vi "Capacitive Message Loop.vi"(8 "error in (no error)":errorcluster, 10 "Data Notifiers":T1, 11 "Message Queues":T2) -> (0 "error out":errorcluster)   [LabVIEW 2013, in "Capacitive.lvlib"]
uses:
  Capacitive.lvlib
  support/Message Queue/All Message Queues.ctl
  support/Message Queue/Message Cluster.ctl
  support/Data Notifiers/All Data Notifiers.ctl
  Acquisition/APD Notifier Cluster.ctl
  Piezo/Piezo display.ctl
  XY/XY Display.ctl
  Capacitive Signal Cluster.ctl
  Hardware Configuration.ctl
  Acquisition/Acquisition State.ctl
  support/Message Queue/Enqueue Message (Single).vi
  <vilib>/Utility/error.llb/Error Cluster From Error Code.vi
  <vilib>/ErrorRing/Error Ring.xnode
  Acquisition/Acquisition.lvlib
  support/Message Queue/Message Queue.lvlib
  Piezo/Piezo.lvlib
  XY/XY.lvlib
  support/Data Notifiers/Data Notifiers.lvlib
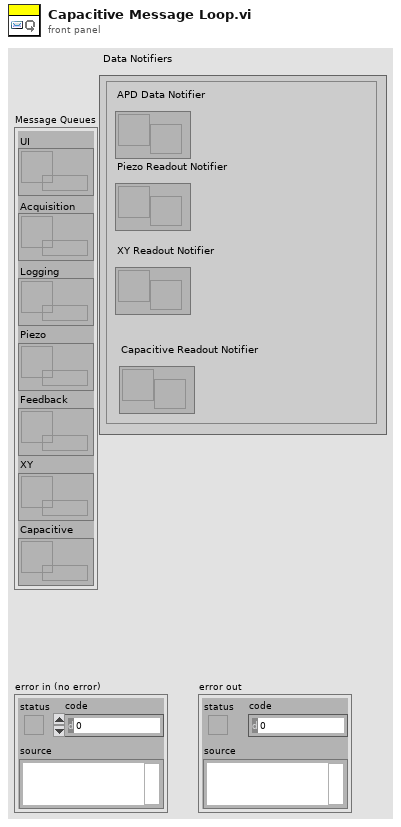
[diagram p1: front panel]
types:
  T1 = typedef "Data Notifiers.lvlib/All Data Notifiers.ctl" = cluster{"APD Data Notifier":refnum<notifier>, "Piezo Readout Notifier":refnum<notifier>, "XY Readout Notifier":refnum<notifier>, "Capacitive Readout Notifier":refnum<notifier>}
  T2 = typedef "Message Queue.lvlib/All Message Queues.ctl" = cluster{"UI":refnum<queue>, "Acquisition":refnum<queue>, "Logging":refnum<queue>, "Piezo":refnum<queue>, "Feedback":refnum<queue>, "XY":refnum<queue>, "Capacitive":refnum<queue>}
  T3 = typedef "Capacitive.lvlib/Hardware Configuration.ctl" = cluster{"IP Address":string, "Handle":u32, "Refresh Time (ms)":dbl}
  T4 = typedef "Acquisition.lvlib/Acquisition State.ctl" = enum16{"Idle", "Acquiring"}
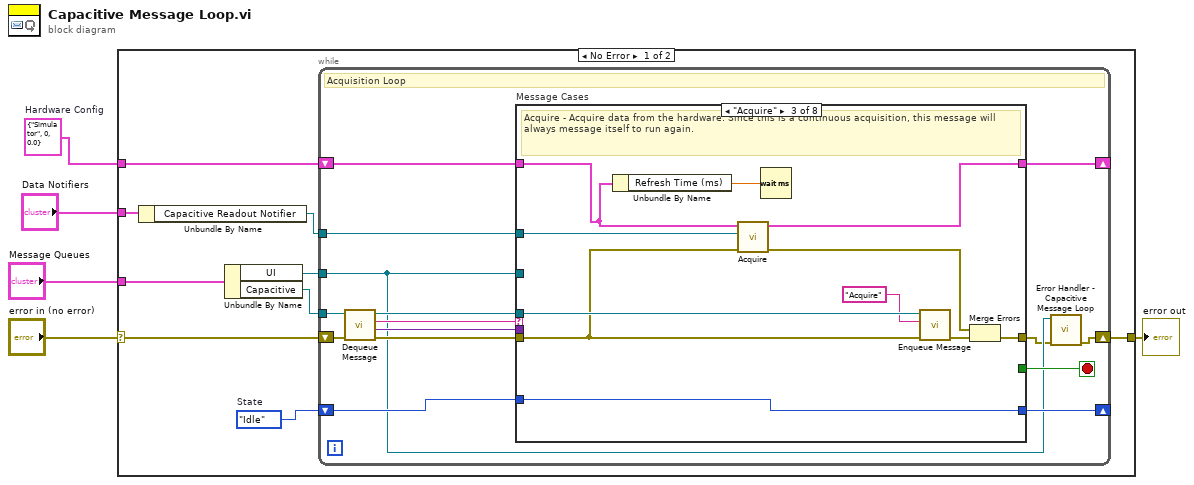
[diagram p0: block diagram]
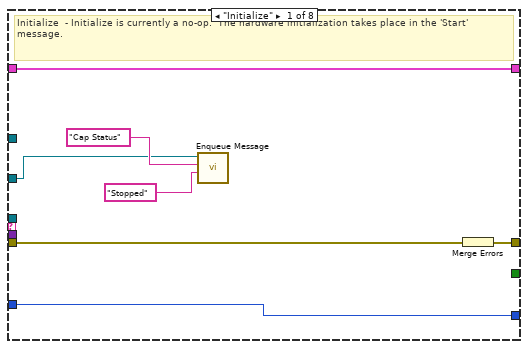
[diagram p2: hidden frame]
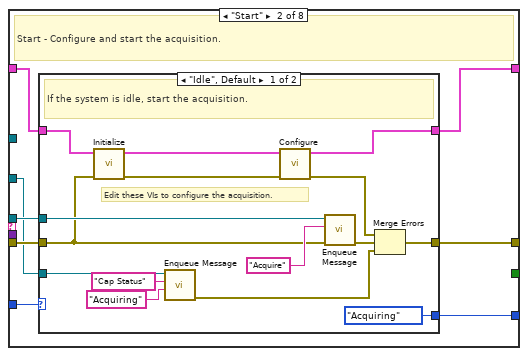
[diagram p3: hidden frame]
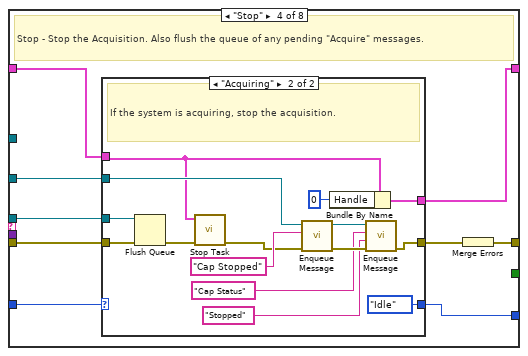
[diagram p5: hidden frame]
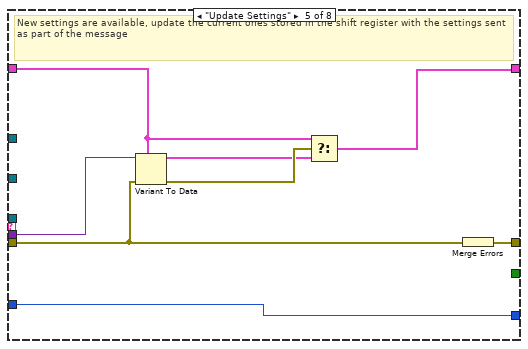
[diagram p7: hidden frame]
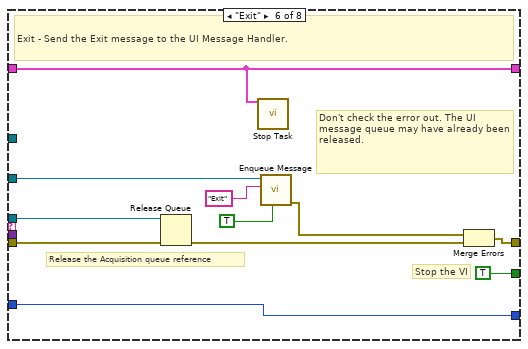
[diagram p8: hidden frame]
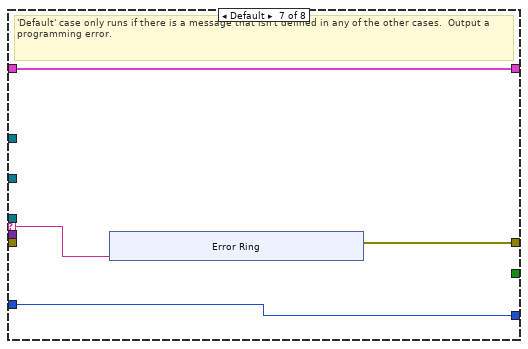
[diagram p9: hidden frame]
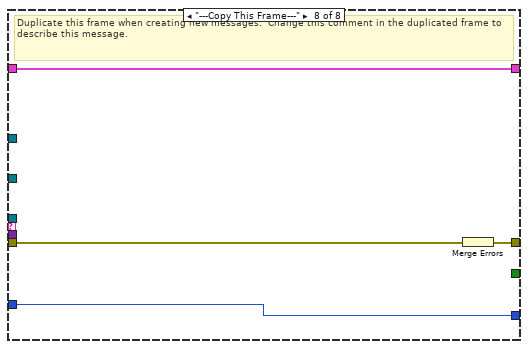
[diagram p10: hidden frame]
diagram:
  w2 = T3 {"IP Address"="Simulator", "Handle"=0, "Refresh Time (ms)"=0.0}  # Hardware Config
  n1 = case shown="No Error" "error in (no error)" {
    selector: "error in (no error)" -> [w11 w135]
    tunnel: "Message Queues" -> [w14 _]
    tunnel: [w12 w135] -> w4
    tunnel: w2 -> [w8 _]
    tunnel: "Data Notifiers" -> [w7 _]
    frame No Error {
      w9 = Acquisition_State."Idle"  # State
      n2 = Unbundle By Name(w7) -> ("Capacitive Readout Notifier"=w6:refnum<notifier>)
      n3 = Unbundle By Name(w14) -> ("UI"=w10:refnum<queue>, "Capacitive"=w13:refnum<queue>)
      n4 = while {
        tunnel: w13 -> [w21]
        shift-right: [w28] -> _
        shift-left: w8 -> [w29]
        shift-right: [w15] -> w12
        shift-left: w11 -> [w26]
        tunnel: w10 -> [w17]
        shift-right: [w19] -> _
        shift-left: w9 -> [w20]
        tunnel: w6 -> [w18]
        stop <- w27 stop-if-true
        # "Acquisition Loop"
        n5 = call "Dequeue Message.vi"("error in (no error)"=w26, "Message Queue"=w21) -> ("error out"=w25:errorcluster, "Message Data"=w23:variant, "Message"=w24:string, "dup Message Queue"=w22:refnum<queue>)  [unwired: 6 in]
        n6 = case "Message Cases" shown="\"Acquire\"" w24 {
          selector: w24 -> [_ _ _ _ _ _ w122 _]
          tunnel: w22 -> [_ w41 w71 w79 _ w112 _ _]
          tunnel: w25 -> [w35 w42 w67 w81 w102 w116 _ w134]
          tunnel: [w36 w44 w73 w82 w108 w118 w121 w132] -> w16
          tunnel: w29 -> [w34 w43 w64 w80 w104 w110 w123 w133]
          tunnel: [w34 w40 w68 w74 w103 w110 w123 w133] -> w28
          tunnel: [_ _ _ _ _ TRUE _ _] -> w27
          tunnel: w23 -> [_ _ _ _ w107 _ _ _]
          tunnel: w17 -> [w30 w37 _ w78 _ w117 _ _]
          tunnel: w20 -> [w33 w39 w69 w77 w101 w111 w120 w131]
          tunnel: [w33 w38 w69 w76 w101 w111 w120 w131] -> w19
          tunnel: w18 -> [_ _ w65 _ _ _ _ _]
          frame "Initialize" {
            # "Initialize  - Initialize is currently a no-op.  The hardware initialization takes place in the 'Start' message."
            n7 = call-poly "Enqueue Message.vi"("Message Data"="Stopped" ("Message"), "Message"="Cap Status", "Message Queue"=w30) -> ()  [unwired: 7 in, 2 out]
            n8 = Merge Errors(w35) -> (w36:errorcluster)
          }
          frame "Start" {
            # "Start - Configure and start the acquisition."
            n9 = case shown="\"Idle\", Default" w39 {
              selector: w39 -> [_ w60]
              tunnel: [w59 w62] -> w44
              tunnel: w43 -> [w53 w61]
              tunnel: w42 -> [w54 w62]
              tunnel: w41 -> [w57 _]
              tunnel: [w51 w61] -> w40
              tunnel: [Acquisition_State."Acquiring" ("State") w60] -> w38
              tunnel: w37 -> [w47 _]
              frame "Idle", Default {
                # "Edit these VIs to configure the acquisition."
                # "If the system is idle, start the acquisition."
                n10 = call "Initialize.vi"("error in (no error)"=w54, "Hardware Refs In"=w53) -> ("error out"=w50:errorcluster, "Hardware Refs Out"=w52:T3)  [unwired: 8 in]
                n11 = call-poly "Enqueue Message.vi"("Message Data"="Acquiring" ("Message"), "Message"="Cap Status", "Message Queue"=w47) -> ("error out"=w48:errorcluster)  [unwired: 7 in, 1 out]
                n12 = call "Configure.vi"("error in (no error)"=w50, "Hardware Refs In"=w52) -> ("error out"=w49:errorcluster, "Hardware Refs Out"=w51:T3)  [unwired: 8 in]
                n13 = call-poly "Enqueue Message.vi"("error in (no error)"=w54, "Message"="Acquire", "Message Queue"=w57) -> ("error out"=w58:errorcluster)  [unwired: 7 in, 1 out]
                n14 = Merge Errors(w49, w58, w48) -> (w59:errorcluster)
              }
              frame "Acquiring" {
                # "The system is already acquiring. Ignore the \"Start\" message."
              }
            }
          }
          frame "Acquire" {
            # "Acquire - Acquire data from the hardware. Since this is a continuous acquisition, this message will always message itself to run again."
            n15 = Unbundle By Name(w64) -> ("Refresh Time (ms)"=w63:dbl)
            n16 = call "Acquire.vi"("error in (no error)"=w67, "Capacitive Readout Notifier"=w65, "Hardware Refs In"=w64) -> ("error out"=w66:errorcluster, "Hardware Refs Out"=w68:T3)  [unwired: 7 in]
            n17 = Wait (ms)(milliseconds to wait=w63) -> ()  [unwired: 1 out]
            n18 = call-poly "Enqueue Message.vi"("error in (no error)"=w67, "Message"="Acquire", "Message Queue"=w71) -> ("error out"=w72:errorcluster)  [unwired: 7 in, 1 out]
            n19 = Merge Errors(w66, w72) -> (w73:errorcluster)
          }
          frame "Stop" {
            # "Stop - Stop the Acquisition. Also flush the queue of any pending \"Acquire\" messages."
            n20 = case shown="\"Acquiring\"" w77 {
              selector: w77 -> [w85 _]
              tunnel: w81 -> [w84 w100]
              tunnel: w80 -> [w83 w93]
              tunnel: w79 -> [_ w99]
              tunnel: w78 -> [_ w98]
              tunnel: [w85 Acquisition_State."Idle" ("State")] -> w76
              tunnel: [w84 w89] -> w75
              tunnel: [w83 w91] -> w74
              frame "Idle", Default {
                # "The system is already idle. Ignore the \"Stop\" message."
              }
              frame "Acquiring" {
                # "If the system is acquiring, stop the acquisition."
                n21 = Flush Queue(queue=w99, error in (no error)=w100) -> (error out=w95:errorcluster)  [unwired: 2 out]
                n22 = call "Stop Task.vi"("error in (no error)"=w95, "Hardware Refs In"=w93) -> ("error out"=w94:errorcluster)  [unwired: 9 in]
                n23 = call-poly "Enqueue Message.vi"("error in (no error)"=w94, "Message"="Cap Stopped", "Message Queue"=w98) -> ("error out"=w90:errorcluster, "dup Message Queue"=w88:refnum<queue>)  [unwired: 7 in]
                n24 = Bundle By Name(cluster=w93, "Handle"=u32 0) -> (w91:T3)
                n25 = call-poly "Enqueue Message.vi"("error in (no error)"=w90, "Message Data"="Stopped" ("Message"), "Message"="Cap Status", "Message Queue"=w88) -> ("error out"=w89:errorcluster)  [unwired: 6 in, 1 out]
              }
            }
            n26 = Merge Errors(w75) -> (w82:errorcluster)
          }
          frame "Update Settings" {
            # "New settings are available, update the current ones stored in the shift register with the settings sent as part of the message"
            n27 = Variant To Data(error in=w102, type=w104, Variant=w107) -> (data=w105:T3, error out=w106:errorcluster)
            n28 = Select(t=w104, s=w106, f=w105) -> (s? t:f=w103:T3)
            n29 = Merge Errors(w102) -> (w108:errorcluster)
          }
          frame "Exit" {
            # "Don't check the error out. The UI message queue may have already been released."
            # "Release the Acquisition queue reference"
            # "Stop the VI"
            # "Exit - Send the Exit message to the UI Message Handler."
            n30 = Release Queue(queue=w112, error in (no error)=w116) -> (error out=w113:errorcluster)  [unwired: 1 in, 2 out]
            n31 = call "Stop Task.vi"("Hardware Refs In"=w110) -> ()  [unwired: 10 in, 1 out]
            n32 = call-poly "Enqueue Message.vi"("Priority Message? (F)"=TRUE, "Message"="Exit", "Message Queue"=w117) -> ("error out"=w109:errorcluster)  [unwired: 7 in, 1 out]
            n33 = Merge Errors(w109, w113) -> (w118:errorcluster)
          }
          frame Default {
            # "'Default' case only runs if there is a message that isn't defined in any of the other cases.  Output a programming error."
            n34 = xnode "Error Ring"("parameter 0"=w122) -> ("error out"=w121:errorcluster)
          }
          frame "---Copy This Frame---" {
            # "Duplicate this frame when creating new messages.  Change this comment in the duplicated frame to describe this message."
            n35 = Merge Errors(w134) -> (w132:errorcluster)
          }
        }
        n36 = call "Error Handler - Capacitive Message Loop.vi"("error in (no error)"=w16, "Message Queue"=w17) -> ("dup error in"=w15:errorcluster)  [unwired: 8 in, 1 out]
      }
    }
    frame Error {
    }
  }
  "error out" <- w4
